vi "EEG Logging (Emotiv Epoc).vi"() -> ()   [LabVIEW 2016]
uses:
  EmotivEpocEEGLogger/_vlib/EE_Queue_Refnum.ctl
  EmotivEpocEEGLogger/_vlib/EE_Queue_Data_Type.ctl
  EmotivEpocEEGLogger/_vlib/EE_SignalStrength_enum.ctl
  EmotivEpocEEGLogger/_vlib/EE_EEG_ContactQuality_enum.ctl
  EmotivEpocEEGLogger/_vlib/EE_Notifier_Refnum.ctl
  EmotivEpocEEGLogger/_vlib/EE_Notifier_Data_Type.ctl
  EmotivEpocEEGLogger/_vlib/EE_EEG_File_Type.ctl
  EmotivEpocEEGLogger/_vlib/EE_ApplicationState.ctl
  EmotivEpocEEGLogger/_vlib/EmotivEpocHeadsetControls.lvclass
  <vilib>/Utility/error.llb/DialogType.ctl
  Emotiv Epoc.lvlib
panel:
  out "NotifierRefnum":T1
  out "QueueRefnum":T2
  in  "Exit Button":bool
  out "Application State":string caption="Состояние"
  in  "Tab Control":enum32{"Начало", "Просмотр ЭЭГ"}(tab)
  in  "EEG_File_Type":T3=enum."TXT"
  in  "Apply Settings":bool
  in  "User name":string caption="Имя пользователя"
  in  "Path to the working folder":path caption="Путь к рабочей папке"
  in  "Path to edk.dll":path caption="Путь к dll-файлу"
  in  "Probe Stop":bool
  in  "Probe Start":bool
  out "O1":bool
  out "P7":bool
  out "CMS":bool
  out "AF4":bool
  out "T7":bool
  out "F8":bool
  out "F4":bool
  out "FC6":bool
  out "T8":bool
  out "DRL":bool
  out "P8":bool
  out "O2":bool
  out "AF3":bool
  out "F3":bool
  out "F7":bool
  out "FC5":bool
  out "Wireless Signal Strength":u32(slide) caption="Качество сигнала" scale=0.0..2.0
  in  "Emotiv Epoc Error Code":string="0000  0" caption="Индикация ошибок"
  out "EEG Waveform Chart":waveform(dbl)[](graph) caption="График ЭЭГ"
  in  "Start Logging":bool
  # "This VI is a part of BCI Design library, http://www.ru-bci.org \nCopyright © 2020, Sotnikov Peter, All rights reserved. License: CC BY-NC 4.0"
  # "Запись ЭЭГ в файлы формата:"
  # "Проба"
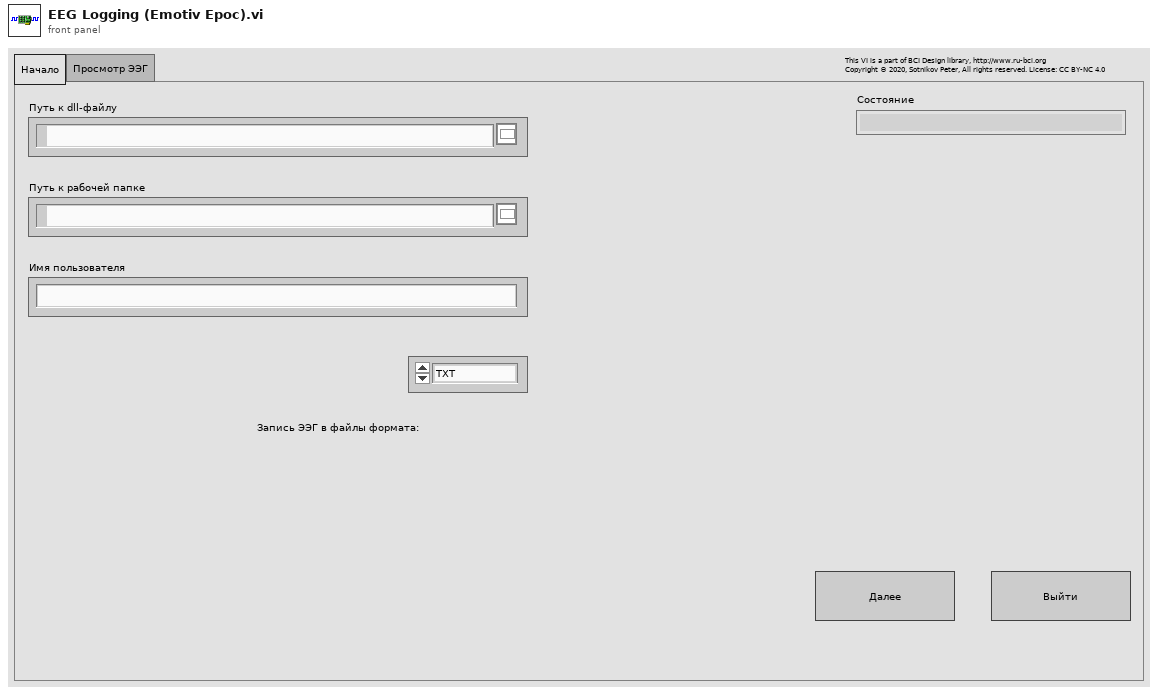
[diagram p1: front panel]
types:
  T1 = typedef "Emotiv Epoc.lvlib/EE_Notifier_Refnum.ctl" = refnum<notifier>
  T2 = typedef "Emotiv Epoc.lvlib/EE_Queue_Refnum.ctl" = refnum<queue>
  T3 = typedef "Emotiv Epoc.lvlib/EE_EEG_File_Type.ctl" = enum16{"XML", "TXT"}
  T4 = typedef "Emotiv Epoc.lvlib/EE_ApplicationState.ctl" = enum16{"Start", "Work", "Stop"}
  T5 = typedef "Emotiv Epoc.lvlib/EE_Notifier_Data_Type.ctl" = cluster{"EDK_Error":string, "Number of samples":u32, "Marker Waveform":waveform(dbl), "Array of EEG waveforms":waveform(dbl)[], "WirelessSignalStatus":T6, "EEG_ContactsQuality":T7[]}
  T6 = typedef "Emotiv Epoc.lvlib/EmotivEpocHeadsetControls.lvclass/EE_SignalStrength_enum.ctl" = enum32{"NO_SIGNAL", "BAD_SIGNAL", "GOOD_SIGNAL"}
  T7 = typedef "Emotiv Epoc.lvlib/EE_EEG_ContactQuality_enum.ctl" = enum16{"EEG_CQ_NO_SIGNAL", "EEG_CQ_VERY_BAD", "EEG_CQ_POOR", "EEG_CQ_FAIR", "EEG_CQ_GOOD"}
  T8 = typedef "Emotiv Epoc.lvlib/EE_Queue_Data_Type.ctl" = cluster{"FinishedLate?":bool, "UserActive?":bool, "WirelessSignalStatus":T6, "EDK_ERROR_CODE":i32, "nSampleOut":u32, "CurrentTimestamp":timestamp, "RawChannelsData ":dbl[][], "EEG_ContactsQuality":T7[]}
  T9 = typedef "DialogType.ctl" = u16
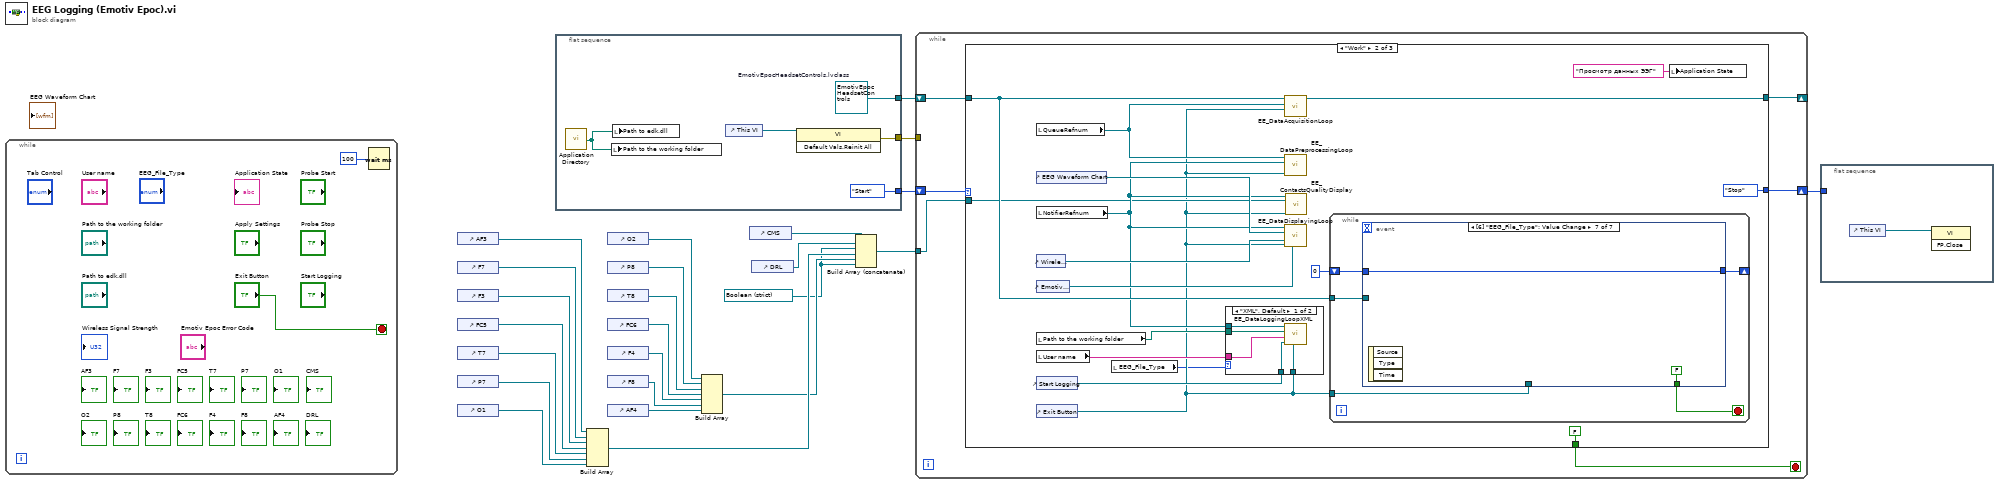
[diagram p0: block diagram]
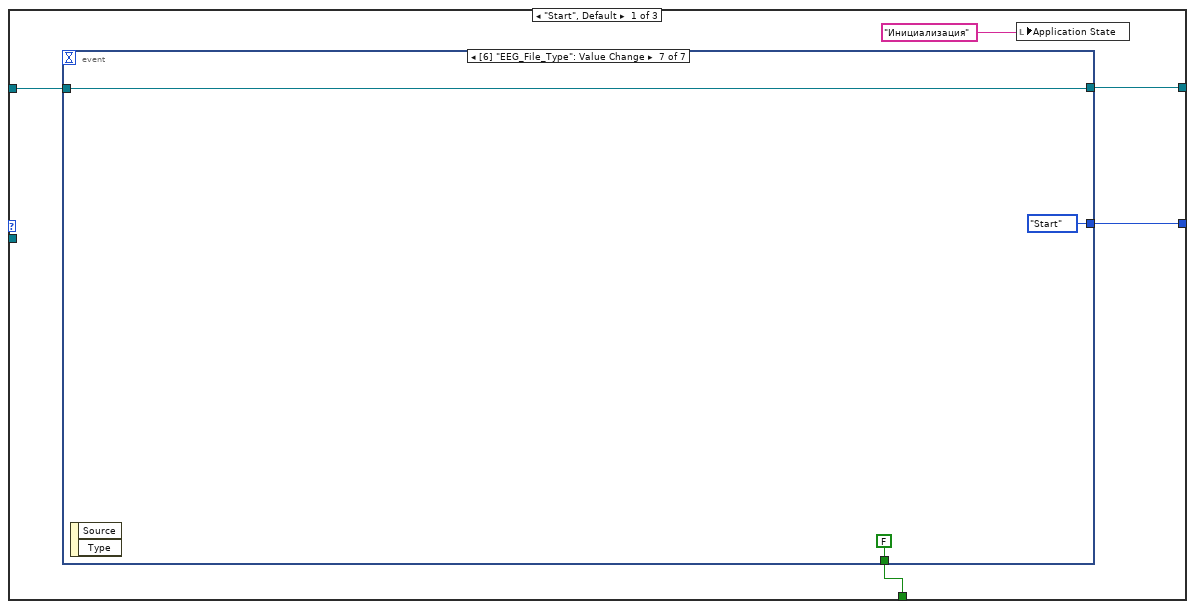
[diagram p2: hidden frame]
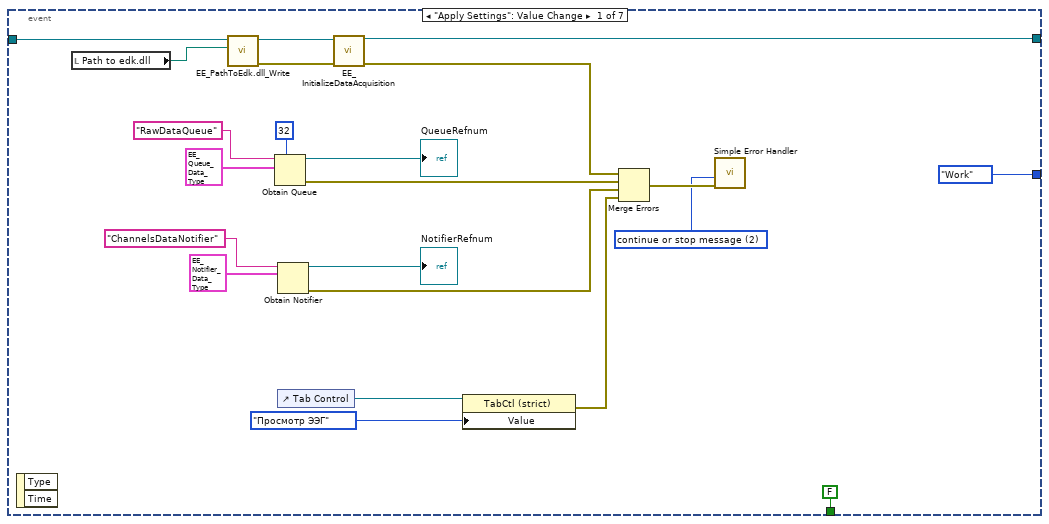
[diagram p3: hidden frame]
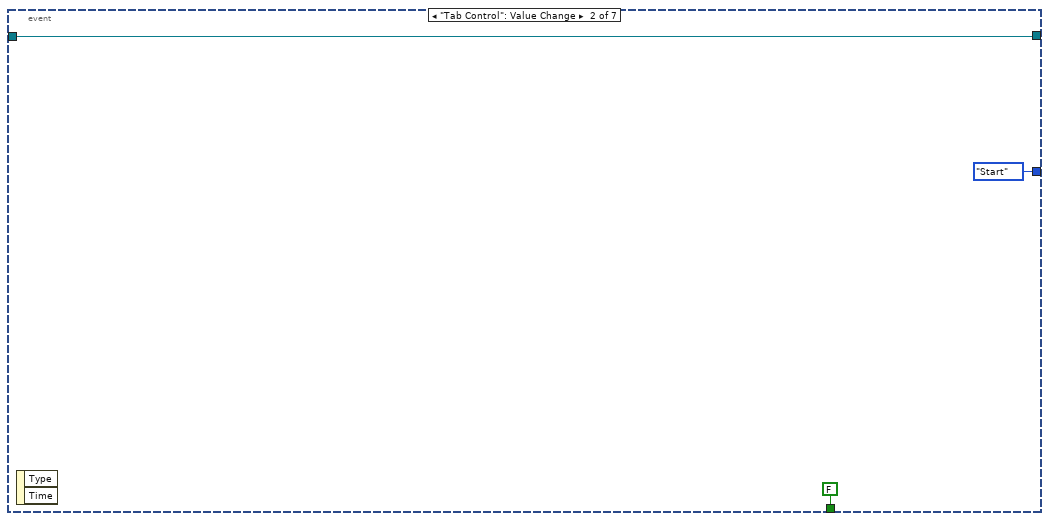
[diagram p4: hidden frame]
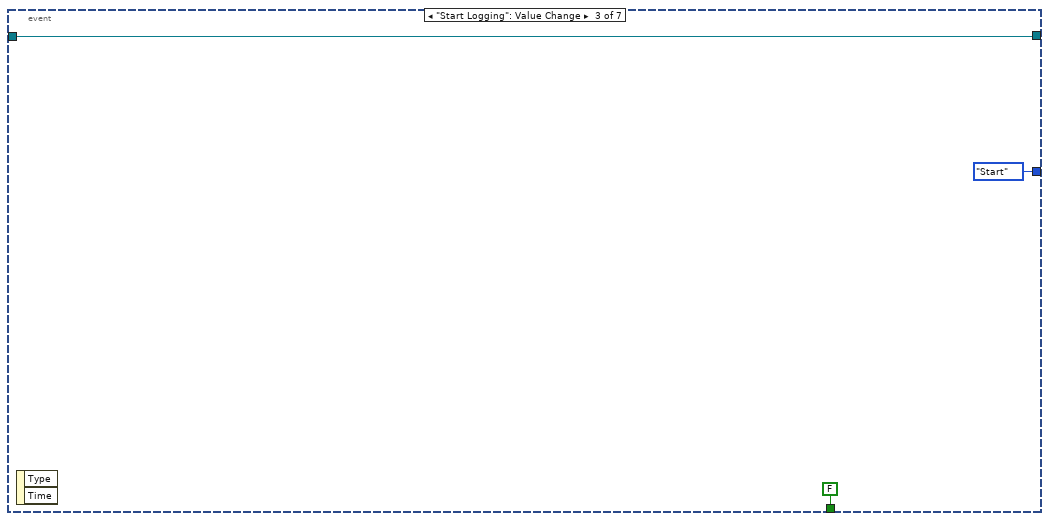
[diagram p5: hidden frame]
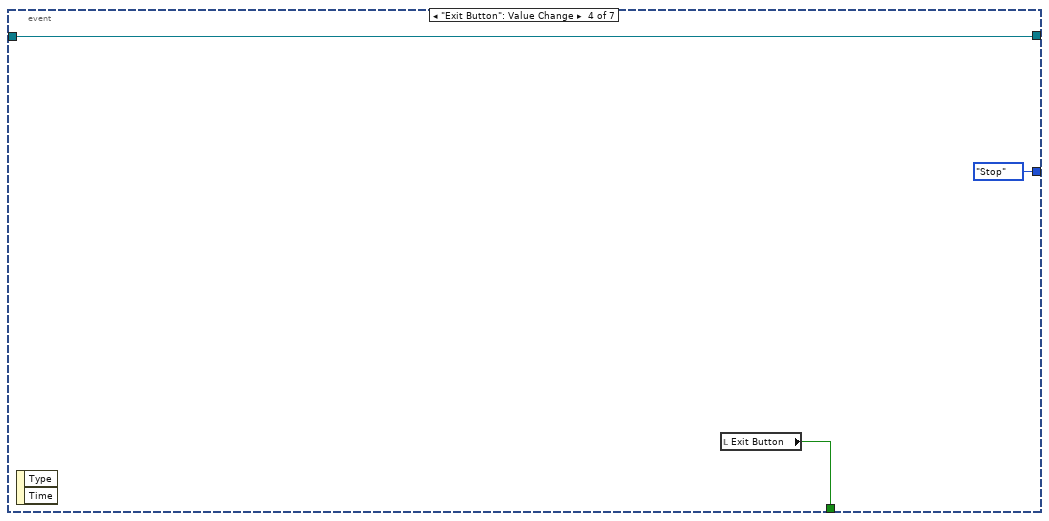
[diagram p6: hidden frame]
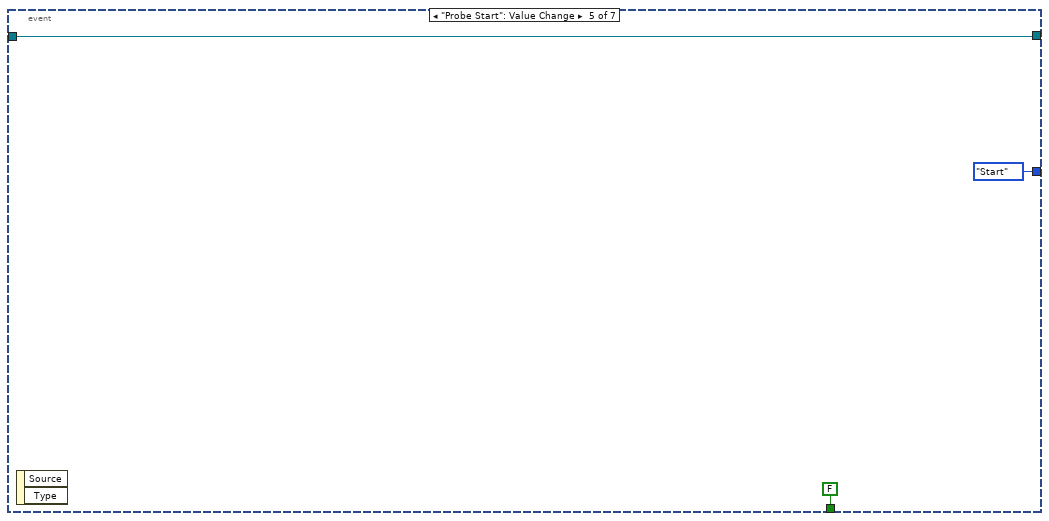
[diagram p7: hidden frame]
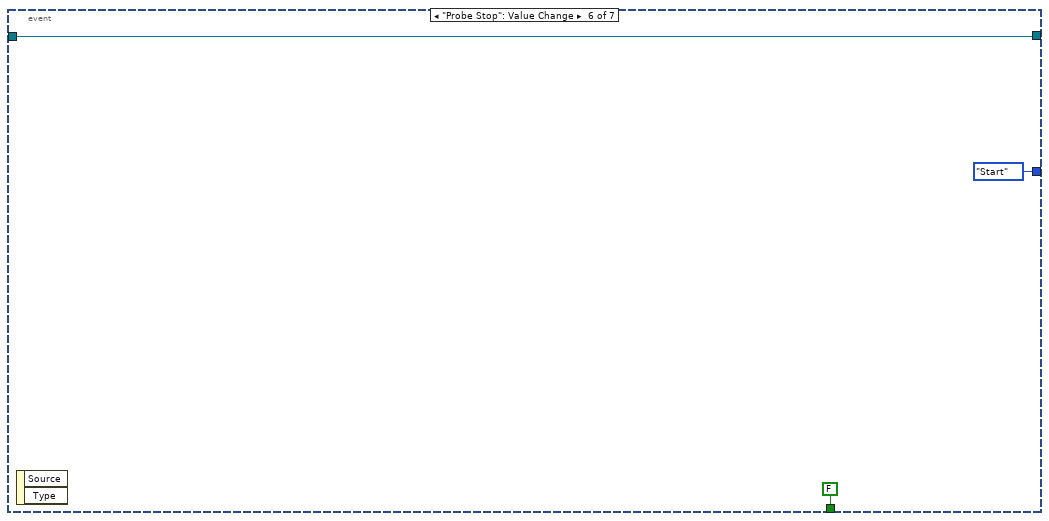
[diagram p8: hidden frame]
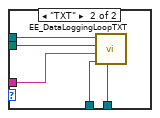
[diagram p9: hidden frame]
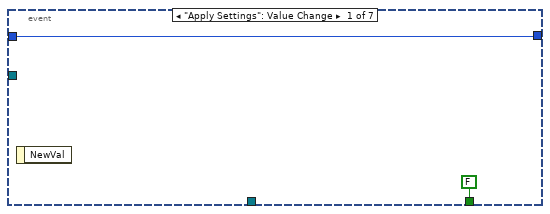
[diagram p10: hidden frame]
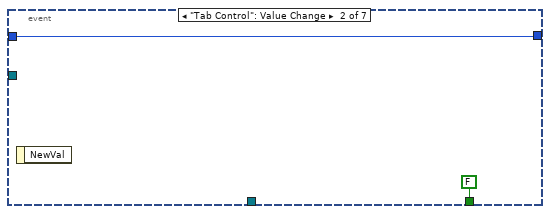
[diagram p11: hidden frame]
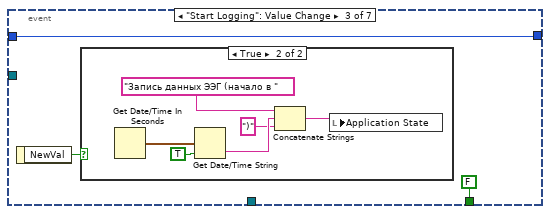
[diagram p12: hidden frame]
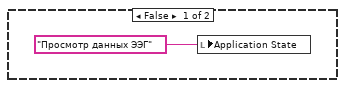
[diagram p13: hidden frame]
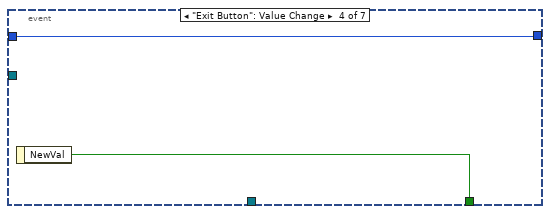
[diagram p14: hidden frame]
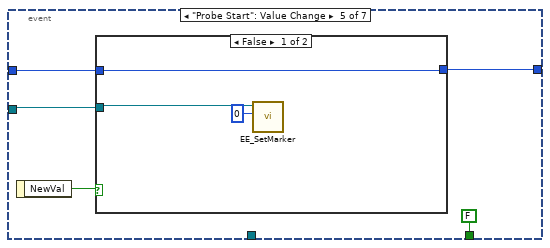
[diagram p15: hidden frame]
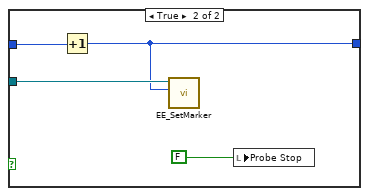
[diagram p16: hidden frame]
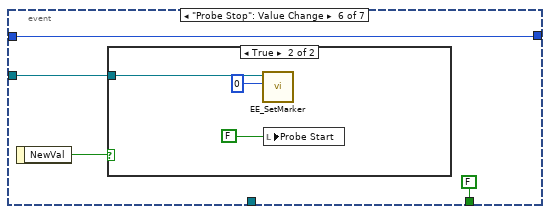
[diagram p17: hidden frame]
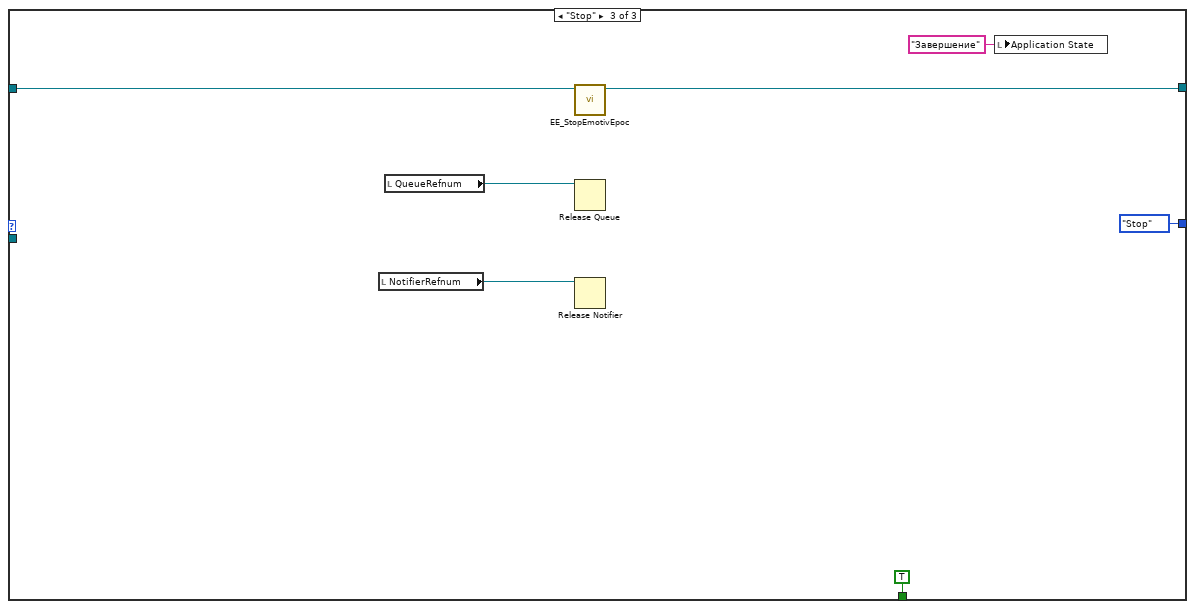
[diagram p19: hidden frame]
diagram:
  w3 = refnum<vi> refnum ("element")
  n1 = while {
    stop <- "Exit Button" stop-if-true
    n2 = Wait (ms)(milliseconds to wait=u32 100) -> ()  [unwired: 1 out]
  }
  n3 = control-ref of="AF3"() -> (w21:refnum<vi>)
  n4 = control-ref of="F7"() -> (w20:refnum<vi>)
  n5 = control-ref of="F3"() -> (w19:refnum<vi>)
  n6 = control-ref of="FC5"() -> (w18:refnum<vi>)
  n7 = control-ref of="T7"() -> (w17:refnum<vi>)
  n8 = control-ref of="P7"() -> (w16:refnum<vi>)
  n9 = control-ref of="O1"() -> (w15:refnum<vi>)
  n10 = flat-sequence {
    tunnel: [EE_ApplicationState."Start" ("ApplicationState")] -> w24
    tunnel: [w30] -> w23
    tunnel: [w28] -> w22
    frame #0 {
      w30 = refnum<class "EmotivEpocHeadsetControls.lvclass"> refnum  # EmotivEpocHeadsetControls.lvclass
      n11 = call <vilib>:"Application Directory.vi"() -> ("Application Directory"=w27:path)
      n12 = local write "Path to the working folder"(w27) -> ()
      n13 = local write "Path to edk.dll"(w27) -> ()
      n14 = control-ref of="This VI"() -> (w29:refnum<vi>)
      n15 = invoke class="VI" method="Default Vals.Reinit All"(reference=w29) -> (error out=w28:errorcluster)  [unwired: 2 in, 2 out]
    }
  }
  n16 = Build Array(w21, w20, w19, w18, w17, w16, w15) -> (w5:refnum<vi>[])
  n17 = control-ref of="O2"() -> (w12:refnum<vi>)
  n18 = control-ref of="P8"() -> (w8:refnum<vi>)
  n19 = control-ref of="T8"() -> (w9:refnum<vi>)
  n20 = control-ref of="FC6"() -> (w10:refnum<vi>)
  n21 = control-ref of="F4"() -> (w11:refnum<vi>)
  n22 = control-ref of="F8"() -> (w13:refnum<vi>)
  n23 = control-ref of="AF4"() -> (w14:refnum<vi>)
  n24 = Build Array(w12, w8, w9, w10, w11, w13, w14) -> (w4:refnum<vi>[])
  n25 = control-ref of="CMS"() -> (w7:refnum<vi>)
  n26 = control-ref of="DRL"() -> (w6:refnum<vi>)
  n27 = Build Array (concatenate)(w7, w6, w3, w5, w4, w3) -> (w2:refnum<vi>[])
  n28 = while {
    shift-right: [w34] -> w1
    shift-left: w24 -> [w37]
    shift-right: [w35] -> _
    shift-left: w23 -> [w36]
    tunnel: w22 -> [_]
    tunnel: w2 -> [w32]
    stop <- w33 stop-if-true
    n29 = case shown="\"Work\"" w37 {
      tunnel: w36 -> [w42 w89 w155]
      tunnel: [w41 w90 w154] -> w35
      tunnel: [w40 EE_ApplicationState."Stop" ("ApplicationState") EE_ApplicationState."Stop" ("ApplicationState")] -> w34
      tunnel: [w39 FALSE ("Stop Button") TRUE ("Stop Button")] -> w33
      tunnel: w32 -> [_ w86 _]
      frame "Start", Default {
        n30 = event shown="[6] \"EEG_File_Type\": Value Change" {
          selector: _ -> [_ _ _ _ _ _ _]
          dyn-events: _ -> [_ _ _ _ _ _ _]
          timeout: _ -> [_ _ _ _ _ _ _]
          tunnel: w42 -> [w50 w67 w70 w73 w76 w78 w82]
          tunnel: [w48 w67 w70 w73 w76 w78 w82] -> w41
          tunnel: [EE_ApplicationState."Work" ("ApplicationState") EE_ApplicationState."Start" ("ApplicationState") EE_ApplicationState."Start" ("ApplicationState") EE_ApplicationState."Stop" ("ApplicationState") EE_ApplicationState."Start" ("ApplicationState") EE_ApplicationState."Start" ("ApplicationState") EE_ApplicationState."Start" ("ApplicationState")] -> w40
          tunnel: [FALSE ("Stop Button") FALSE ("Stop Button") FALSE ("Stop Button") w71 FALSE ("Stop Button") FALSE ("Stop Button") FALSE ("Stop Button")] -> w39
          event "Apply Settings": Value Change {
            w52 = T9 2 items=["no dialog", "OK message", "continue or stop message", "OK message + warnings", "continue/stop + warnings"] ("type of dialog (OK msg:1)")
            n31 = event-data() -> ()  [unwired: 1 in, 2 out]
            n32 = local read "Path to edk.dll"() -> (w49:path)
            n33 = call-dynamic "EE_PathToEdk.dll_Write.vi"("PathToEdk.dll"=w49, "EmotivEpocHeadsetControls in"=w50) -> ("error out"=w64:errorcluster, "EmotivEpocHeadsetControls out"=w63:refnum<class "EmotivEpocHeadsetControls.lvclass">)  [unwired: 8 in]
            n34 = Obtain Queue(max queue size (-1, unlimited)=32, name (unnamed)="RawDataQueue", element data type=T8 {"FinishedLate?"=FALSE, "UserActive?"=FALSE, "WirelessSignalStatus"=enum."NO_SIGNAL", "EDK_ERROR_CODE"=0, "nSampleOut"=0, "CurrentTimestamp"=timestamp(0 s since 1904-01-01), "RawChannelsData "=[], "EEG_ContactsQuality"=[]} ("Queue_Data_Type")) -> (queue out=→"QueueRefnum":refnum<queue>, error out=w56:errorcluster)  [unwired: 2 in, 1 out]
            n35 = Obtain Notifier(name (unnamed)="ChannelsDataNotifier", notification data type=T5 {"EDK_Error"="No data received. Check your device", "Number of samples"=0, "Marker Waveform"={"t0"=timestamp(0 s since 1904-01-01), "dt"=1.0, "Y"=[]}, "Array of EEG waveforms"=[], "WirelessSignalStatus"=enum."NO_SIGNAL", "EEG_ContactsQuality"=[]} ("Notifier Data Type")) -> (notifier out=→"NotifierRefnum":refnum<notifier>, error out=w55:errorcluster)  [unwired: 2 in, 1 out]
            n36 = control-ref of="Tab Control"() -> (w47:refnum<vi>)
            n37 = call-dynamic "EE_InitializeDataAcquisition.vi"("EmotivEpocHeadsetControls in"=w63, "error in (no error)"=w64) -> ("EmotivEpocHeadsetControls out"=w48:refnum<class "EmotivEpocHeadsetControls.lvclass">, "error out"=w54:errorcluster)  [unwired: 12 in]
            n38 = property class="TabCtl (strict)"(reference=w47, "Value"=enum32{"Начало", "Просмотр ЭЭГ"}."Просмотр ЭЭГ") -> (error out=w46:errorcluster)  [unwired: 1 in, 1 out]
            n39 = Merge Errors(w54, w56, w55, w46) -> (w53:errorcluster)
            n40 = call <vilib>:"Simple Error Handler.vi"("type of dialog (OK msg:1)"=w52, "error in (no error)"=w53) -> ()  [unwired: 3 in, 5 out]
          }
          event "Tab Control": Value Change {
            n41 = event-data() -> ()  [unwired: 1 in, 2 out]
          }
          event "Start Logging": Value Change {
            n42 = event-data() -> ()  [unwired: 1 in, 2 out]
          }
          event "Exit Button": Value Change {
            n43 = event-data() -> ()  [unwired: 1 in, 2 out]
            n44 = local read "Exit Button"() -> (w71:bool)
          }
          event "Probe Start": Value Change {
            n45 = event-data() -> ()  [unwired: 1 in, 2 out]
          }
          event "Probe Stop": Value Change {
            n46 = event-data() -> ()  [unwired: 1 in, 2 out]
          }
          event Value Change {
            n47 = event-data() -> ()  [unwired: 1 in, 2 out]
          }
        }
        n48 = local write "Application State"("Инициализация" ("Application State")) -> ()
      }
      frame "Work" {
        n49 = local read "QueueRefnum"() -> (w97:T2)
        n50 = control-ref of="EEG Waveform Chart"() -> (w95:refnum<vi>)
        n51 = local read "NotifierRefnum"() -> (w87:T1)
        n52 = control-ref of="Wireless Signal Strength"() -> (w94:refnum<vi>)
        n53 = control-ref of="Emotiv Epoc Error Code"() -> (w96:refnum<vi>)
        n54 = local read "Path to the working folder"() -> (w93:path)
        n55 = local read "User name"() -> (w92:string)
        n56 = control-ref of="Start Logging"() -> (w91:refnum<vi>)
        n57 = control-ref of="Exit Button"() -> (w85:refnum<vi>)
        n58 = local read "EEG_File_Type"() -> (w83:T3)
        n59 = case shown="\"XML\", Default" w83 {
          tunnel: w93 -> [w104 w109]
          tunnel: w92 -> [w103 w108]
          tunnel: w91 -> [w102 w107]
          tunnel: w87 -> [w101 w106]
          tunnel: w85 -> [w100 w105]
          frame "XML", Default {
            n60 = call "EE_DataLoggingLoopXML.vi"("StopButton Refnum"=w100, "EEG Record Refnum"=w102, "UserName"=w103, "Logs directory path"=w104, "ChannelsDataNotifier in"=w101) -> ()  [unwired: 6 in, 1 out]
          }
          frame "TXT" {
            n61 = call "EE_DataLoggingLoopTXT.vi"("StopButton Refnum"=w105, "EEG Record Refnum"=w107, "UserName"=w108, "Logs directory path"=w109, "ChannelsDataNotifier in"=w106) -> ()  [unwired: 6 in, 1 out]
          }
        }
        n62 = call-dynamic "EE_DataAcquisitionLoop.vi"("StopButton Ref"=w85, "RawDataQueue in"=w97, "EmotivEpocHeadsetControls in"=w89) -> ("EmotivEpocHeadsetControls out"=w90:refnum<class "EmotivEpocHeadsetControls.lvclass">)  [unwired: 6 in, 2 out]
        n63 = call "EE_DataPreprocessingLoop.vi"("StopButton Refnum"=w85, "ChannelsDataNotifier in"=w87, "RawChannelsDataQueue in"=w97) -> ()  [unwired: 7 in, 2 out]
        n64 = call "EE_DataDisplayingLoop.vi"("ChannelsDataNotifier in"=w87, "EEG Waveform Chart Refnum"=w95, "Wireless Signal Strength"=w94, "StopButton Refnum"=w85, "Error Message Refnum"=w96) -> ()  [unwired: 9 in, 2 out]
        n65 = call "EE_ContactsQualityDisplay.vi"("ChannelsDataNotifier in"=w87, "Contacts Quality Indicators"=w86, "StopButton Refnum"=w85) -> ()  [unwired: 11 in, 2 out]
        n66 = while {
          tunnel: w89 -> [w114]
          tunnel: w85 -> [w113]
          shift-right: [w110] -> _
          shift-left: 0 ("Marker Value") -> [w111]
          stop <- w112 stop-if-true
          n67 = event shown="[6] \"EEG_File_Type\": Value Change" {
            selector: _ -> [_ _ _ _ _ _ _]
            dyn-events: _ -> [_ _ _ _ _ _ _]
            timeout: _ -> [_ _ _ _ _ _ _]
            tunnel: w114 -> [_ _ _ _ w133 w144 _]
            tunnel: w113 -> [_ _ _ _ _ _ _]
            tunnel: [FALSE ("NewVal") FALSE ("NewVal") FALSE ("NewVal") w130 FALSE ("NewVal") FALSE ("NewVal") FALSE ("NewVal")] -> w112
            tunnel: w111 -> [w115 w117 w120 w129 w132 w143 w151]
            tunnel: [w115 w117 w120 w129 w131 w143 w151] -> w110
            event "Apply Settings": Value Change {
              n68 = event-data() -> ()  [unwired: 1 in, 1 out]
            }
            event "Tab Control": Value Change {
              n69 = event-data() -> ()  [unwired: 1 in, 1 out]
            }
            event "Start Logging": Value Change {
              n70 = event-data() -> ("NewVal"=w119:bool)  [unwired: 1 in]
              n71 = case shown="True" w119 {
                frame False {
                  n72 = local write "Application State"("Просмотр данных ЭЭГ" ("Application State")) -> ()
                }
                frame True {
                  n73 = Get Date/Time In Seconds() -> (seconds since 1Jan1904=w123:timestamp)
                  n74 = Get Date/Time String(seconds (now)=w123, want seconds? (F)=TRUE) -> (time string=w125:string)  [unwired: 1 in, 1 out]
                  n75 = Concatenate Strings("Запись данных ЭЭГ (начало в " ("Application State"), w125, ")" ("string")) -> (w127:string)
                  n76 = local write "Application State"(w127) -> ()
                }
              }
            }
            event "Exit Button": Value Change {
              n77 = event-data() -> ("NewVal"=w130:bool)  [unwired: 1 in]
            }
            event "Probe Start": Value Change {
              n78 = event-data() -> ("NewVal"=w134:bool)  [unwired: 1 in]
              n79 = case shown="False" w134 {
                tunnel: w133 -> [w137 w142]
                tunnel: w132 -> [w138 w141]
                tunnel: [w138 w139] -> w131
                frame False {
                  n80 = call-dynamic "EE_SetMarker.vi"("Marker Value"=0, "EmotivEpocHeadsetControls in"=w137) -> ()  [unwired: 8 in, 2 out]
                }
                frame True {
                  n81 = Increment(x=w141) -> (x+1=w139:i32)
                  n82 = call-dynamic "EE_SetMarker.vi"("Marker Value"=w139, "EmotivEpocHeadsetControls in"=w142) -> ()  [unwired: 8 in, 2 out]
                  n83 = local write "Probe Stop"(FALSE ("Probe Stop")) -> ()
                }
              }
            }
            event "Probe Stop": Value Change {
              n84 = event-data() -> ("NewVal"=w145:bool)  [unwired: 1 in]
              n85 = case shown="True" w145 {
                tunnel: w144 -> [_ w149]
                frame False {
                }
                frame True {
                  n86 = call-dynamic "EE_SetMarker.vi"("Marker Value"=0, "EmotivEpocHeadsetControls in"=w149) -> ()  [unwired: 8 in, 2 out]
                  n87 = local write "Probe Start"(FALSE ("Probe Start")) -> ()
                }
              }
            }
            event Value Change {
              n88 = event-data() -> ()  [unwired: 1 in, 3 out]
            }
          }
        }
        n89 = local write "Application State"("Просмотр данных ЭЭГ" ("Application State")) -> ()
      }
      frame "Stop" {
        n90 = local read "NotifierRefnum"() -> (w156:T1)
        n91 = local read "QueueRefnum"() -> (w157:T2)
        n92 = call-dynamic "EE_StopEmotivEpoc.vi"("EmotivEpocHeadsetControls in"=w155) -> ("EmotivEpocHeadsetControls out"=w154:refnum<class "EmotivEpocHeadsetControls.lvclass">)  [unwired: 9 in, 1 out]
        n93 = Release Queue(queue=w157) -> ()  [unwired: 2 in, 3 out]
        n94 = Release Notifier(notifier=w156) -> ()  [unwired: 2 in, 3 out]
        n95 = local write "Application State"("Завершение" ("Application State")) -> ()
      }
    }
  }
  n96 = flat-sequence {
    tunnel: w1 -> [_]
    frame #0 {
      n97 = control-ref of="This VI"() -> (w159:refnum<vi>)
      n98 = invoke class="VI" method="FP.Close"(reference=w159) -> ()  [unwired: 2 in, 3 out]
    }
  }
